vi "IsTimerDoneSubVI.vi"(0 "End Time (Seconds)":dbl) -> (6 "Time Done":bool, 9 "Time Left":dbl)   [LabVIEW 2019, in "Chapter4-Example1-Library.lvlib"]
uses:
  Chapter4-Example1-Library.lvlib
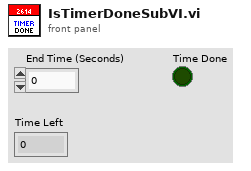
[diagram p1: front panel]
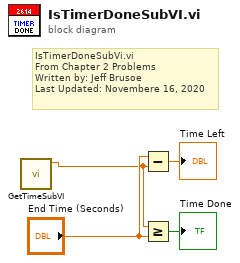
[diagram p0: block diagram]
diagram:
  # "IsTimerDoneSubVi.vi\nFrom Chapter 2 Problems\nWritten by: Jeff Brusoe\nLast Updated: Novembere 16, 2020"
  n1 = call "GetTimeSubVI.vi"() -> ("Seconds"=w1:dbl)  [unwired: 11 in]
  n2 = Subtract(x="End Time (Seconds)", y=w1) -> (x-y=→"Time Left":dbl)
  n3 = Greater Or Equal?(x=w1, y="End Time (Seconds)") -> (x >= y?=→"Time Done":bool)
